vi "viewer.vi"(2 "in":dbl[](array[numeric]), 4 "f_s":dbl) -> (0 "Time-Domain":waveform(dbl)(graph), 1 "Spectrum":cluster{"f0":dbl, "df":dbl, "magnitude":dbl[]}(graph))   [LabVIEW 2017]
uses:
  <vilib>/express/express analysis/Spectral/Block/exnSpectralBlock spectral measurements peak poly.vi
  <vilib>/express/express analysis/Spectral/Block/exnSpectralBlock spectral measurements peak WFM.vi
  <vilib>/express/express analysis/Spectral/XNode/ExpressSpectralMeasurementsBlockNode.xnode
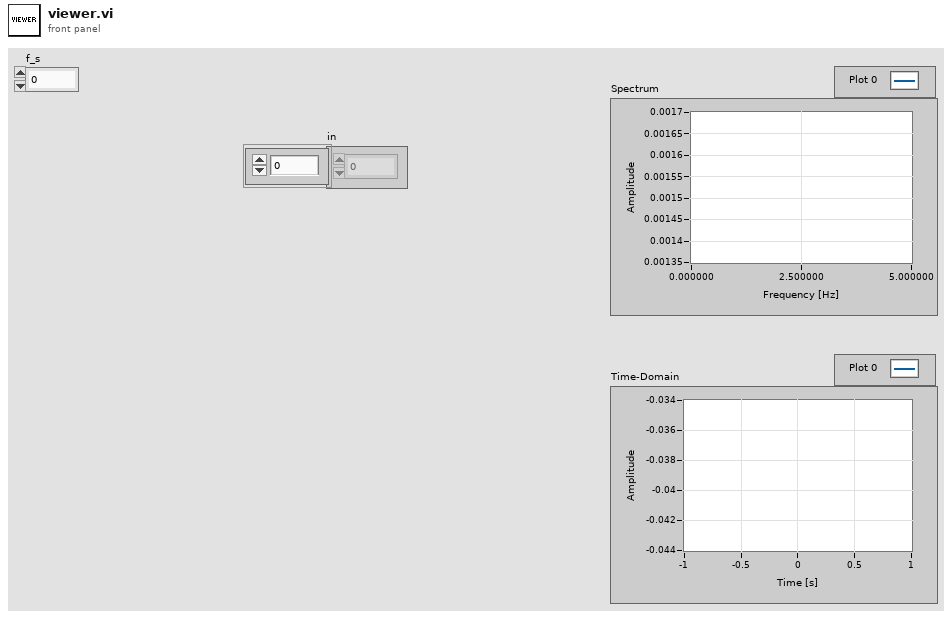
[diagram p1: front panel]
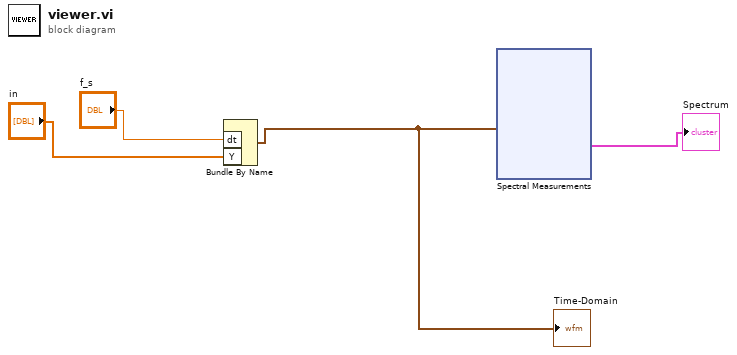
[diagram p0: block diagram]
diagram:
  n1 = Bundle By Name("dt"="f_s", "Y"="in") -> (w2:waveform(dbl))  [unwired: 1 in]
  "Time-Domain" <- w2
  n2 = xnode "Spectral Measurements"("Signals"=w2) -> ("FFT - (Peak)"=→"Spectrum":cluster{"f0":dbl, "df":dbl, "magnitude":dbl[]})  [unwired: 1 in, 2 out]
